vi "contains.vi"(0 "reference":refnum<class "ImplicitParameterNode.lvclass">, 1 "point2D":T1 {"y" format="%.2f"; "x" format="%.2f"}, 2 "AdditionalMargin":i32, 5 "error in (no error)":errorcluster) -> (14 "reference out":refnum<class "ImplicitParameterNode.lvclass">, 15 "contains":bool, 19 "error out":errorcluster)   [LabVIEW 2012, in "ImplicitParameterNode.lvclass"]
doc: "public boolean contains(Point2D p)"
uses:
  <resource>/Framework/Providers/Open_GDS/UML/ImplicitParameterNode_class/ImplicitParameterNode.lvclass
  <resource>/Framework/Providers/Open_GDS/UML/General/Point/Point Point2D.ctl
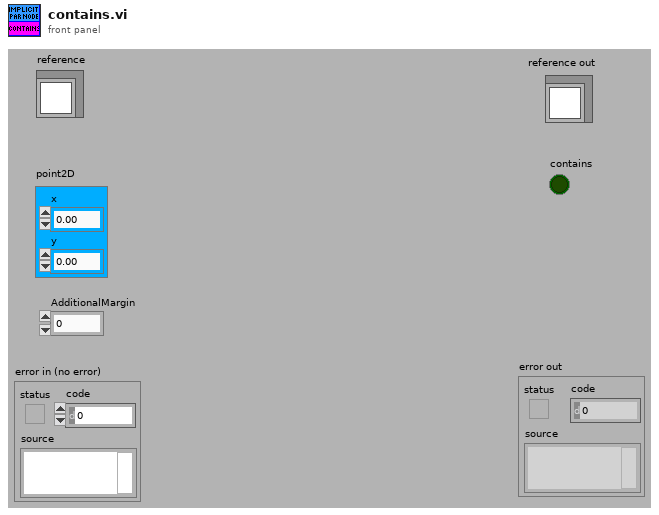
[diagram p1: front panel]
types:
  T1 = typedef "Point Point2D.ctl" = cluster{"x":dbl, "y":dbl}
  T2 = typedef "ImplicitParameterNode.lvclass/ObjectAttributes.ctl" = cluster{"Base class":T3, "topHeight":dbl, "name":refnum<class "MultiLineString.lvclass">, "DEFAULT_TOP_HEIGHT":i32, "DEFAULT_WIDTH":i32, "DEFAULT_HEIGHT":i32}
  T3 = typedef "RectangularNode.lvclass/ObjectAttributes.ctl" = cluster{"Base class":T4, "bounds":T5}
  T4 = typedef "AbstractNode.lvclass/ObjectAttributes.ctl" = cluster{"parent":refnum<class "AbstractNode.lvclass">, "children":refnum<class "AbstractNode.lvclass">[], "Hidden":bool}
  T5 = typedef "Rectangle Rectangle2D.ctl" = cluster{"x":dbl, "y":dbl, "width":dbl, "height":dbl}
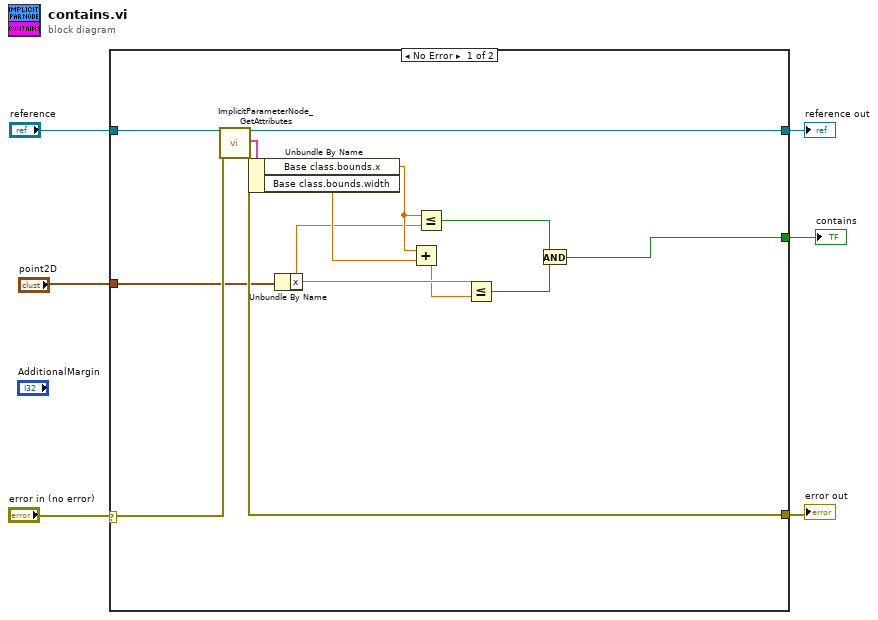
[diagram p0: block diagram]
diagram:
  n1 = case shown="No Error" "error in (no error)" {
    selector: "error in (no error)" -> [w16 w20]
    tunnel: "reference" -> [w19 w21]
    tunnel: [w18 w20] -> w5
    tunnel: [w17 w21] -> w4
    tunnel: [w15 _] -> w2
    tunnel: "point2D" -> [w14 _]
    frame No Error {
      n2 = call <resource>:"ImplicitParameterNode_GetAttributes.vi"("reference in"=w19, "error in (no error)"=w16) -> ("reference out"=w17:refnum<class "ImplicitParameterNode.lvclass">, "Attributes"=w13:T2, "error out"=w18:errorcluster)  [unwired: 15 out]
      n3 = Unbundle By Name(w13) -> ("Base class.bounds.x"=w12:dbl, "Base class.bounds.width"=w11:dbl)
      n4 = Unbundle By Name(w14) -> ("x"=w10:dbl)
      n5 = Add(x=w12, y=w11) -> (x+y=w9:dbl)
      n6 = Less Or Equal?(x=w12, y=w10) -> (x <= y?=w8:bool)
      n7 = Less Or Equal?(x=w10, y=w9) -> (x <= y?=w7:bool)
      n8 = And(x=w8, y=w7) -> (x .and. y?=w15:bool)
    }
    frame Error {
    }
  }
  "reference out" <- w4
  "error out" <- w5
  "contains" <- w2
